vi "v2.vi"() -> ()   [LabVIEW 2024]
uses:
  <vilib>/MakerHub/LINX/LMH-LINX.lvlib
  <vilib>/MakerHub/LINX/Private/Device/Type Defs/Stimulus Pulse.ctl
  <vilib>/MakerHub/LINX/Private/Device/Device.lvlib
  <vilib>/MakerHub/LINX/Public/Utilities/Open Serial.vi
  <vilib>/MakerHub/LINX/Public/Peripherals/Analog/Analog Read 1 Chan.vi
panel:
  in  "Analog Port":u8
  out "Infrared Analog Sinal":dbl(slide) scale=0.0..6.0
  in  "?":bool
  out "Distance (Cm)":dbl(slide) scale=0.0..50.0
  in  "Echo":u8
  in  "Trigger":u8
  in  "Serial Port":refnum<visa-resource-name>="N/A"
  # "This program presents tests conducted with ultrasonic and infrared sensors using the Arduino as a microcontroller. It was developed at the Applied Control Laboratory (LCA) of the Federal Institute of São Paulo by student Guilherme Tinoco. The goal is to evaluate the functionality and accuracy of these sensors."
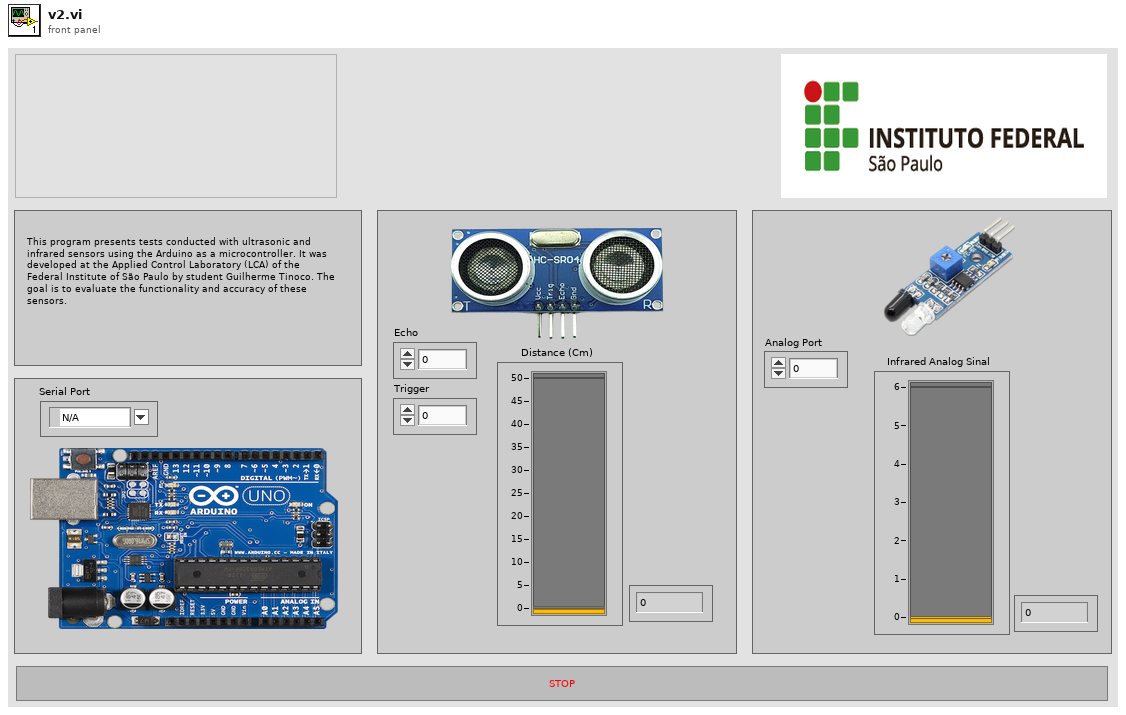
[diagram p1: front panel]
types:
  T1 = typedef "LMH-LINX.lvlib/LINX Ref.ctl" = cluster{"IO":T2, "Interface":T3, "LINX Device Config":T4}
  T2 = typedef "LMH-LINX.lvlib/Platform.ctl" = enum16{"Remote", "Local"}
  T3 = typedef "LMH-LINX.lvlib/Interface.ctl" = enum16{"Serial", "TCP"}
  T4 = typedef "LMH-LINX.lvlib/Device.lvlib/LINX Device Config.ctl" = cluster{"Interface":T3, "COM Port":refnum<visa-resource-name>, "TCP Configuration":T5, "Device Family":u8, "Device ID":u8, "Device Name":string, "TCP Ref":refnum<k5>, "Channels":T6}
  T5 = typedef "LMH-LINX.lvlib/Device.lvlib/TCP Config.ctl" = cluster{"IP Address":string, "Port":u16}
  T6 = typedef "LMH-LINX.lvlib/Channels.ctl" = cluster{"DI":u8[], "DO":u8[], "AI":u8[], "AO":u8[], "PWM":u8[], "QE":u8[], "UART":u8[], "I2C 2":u8[], "SPI":u8[], "CAN":u8[], "Servo":u8[], "AI Ref (V)":dbl, "AI Resolution (Bits)":u8, "AO Ref (V)":dbl, "AO Resolution (Bits)":u8}
  T7 = typedef "LMH-LINX.lvlib/Device.lvlib/Stimulus Pulse.ctl" = enum16{"None", "Active Low", "Active High"}
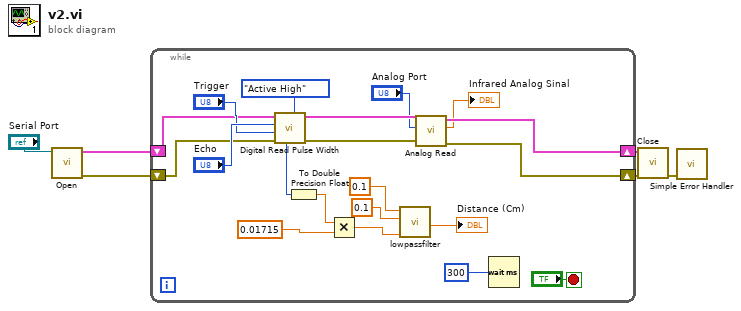
[diagram p0: block diagram]
diagram:
  n1 = call-poly <vilib>:"Open.vi"("Serial Port"="Serial Port") -> ("Error Out"=w4:errorcluster, "LINX Resource"=w6:T1)  [unwired: 8 in, 1 out]
  n2 = while {
    shift-right: [w15] -> w5
    shift-left: w6 -> [w18]
    shift-right: [w13] -> w3
    shift-left: w4 -> [w17]
    stop <- "?" stop-if-true
    n3 = call <vilib>:"Digital Read Pulse Width.vi"("Stimulus Pulse (Active High)"=Stimulus_Pulse."Active High", "Error In"=w17, "DO Channel"="Trigger", "DI Channel"="Echo", "LINX Resource"=w18) -> ("Error Out"=w14:errorcluster, "Pulse Width (uS)"=w19:u32, "LINX Resource"=w16:T1)  [unwired: 4 in]
    n4 = To Double Precision Float(number=w19) -> (double precision float=w26:dbl)
    n5 = Multiply(x=w26, y=0.01715) -> (x*y=w10:dbl)
    n6 = call "lowpassfilter.vi"("In_k"=w10, "Ts"=0.1, "Tf"=0.1) -> ("Filter Output"=→"Distance (Cm)":dbl)  [unwired: 8 in]
    n7 = call-poly <vilib>:"Analog Read.vi"("Error In"=w14, "Analog Channel"="Analog Port", "LINX Resource"=w16) -> ("Error Out"=w13:errorcluster, "Voltage"=→"Infrared Analog Sinal":dbl, "LINX Resource"=w15:T1)  [unwired: 5 in, 1 out]
    n8 = Wait (ms)(milliseconds to wait=u32 300) -> ()  [unwired: 1 out]
  }
  n9 = call <vilib>:"Close.vi"("Error In"=w3, "LINX Resource"=w5) -> ("Error Out"=w1:errorcluster)  [unwired: 9 in]
  n10 = call <vilib>:"Simple Error Handler.vi"("error in (no error)"=w1) -> ()  [unwired: 4 in, 5 out]
